vi "labbbbb.vi"() -> ()   [LabVIEW 2012]
uses:
  <vilib>/imath/engines/lvmath/Plug In/_Char/NIMS_CH_character datatype.ctl
  <vilib>/imath/engines/lvmath2/RunTimeEngine/ErrorHandling/NIMS_Finalize Error.vi
  <vilib>/imath/engines/lvmath2/RunTimeEngine/Managers/WorkSpace/UID Generator.vi
  <vilib>/imath/engines/lvmath2/RunTimeEngine/BuiltInFunctions/length/NIMS_length(GV).vi
  <instcachedir>/0/NIMS_length(GV)_08A3D13377FD4E4B96F5795FBF3698FA.lvgen/NIMS_length(GV)_08A3D13377FD4E4B96F5795FBF3698FA_002.vi
  <vilib>/imath/engines/lvmath2/RunTimeEngine/Managers/SymbolTable/Clear UID.vi
  <vilib>/imath/engines/lvmath2/RunTimeEngine/NodeEndStatement/NIMS_NodeEndStatement_Output.vi
  <instcachedir>/0/NIMS_NodeEndStatement_Output_53EC0D466D134D7ABD903AC30B43404B.lvgen/NIMS_NodeEndStatement_Output_53EC0D466D134D7ABD903AC30B43404B_011.vi
  <vilib>/imath/engines/lvmath2/RunTimeEngine/BuiltInFunctions/linramp/NIMS_linramp.vi
  <vilib>/imath/engines/lvmath2/RunTimeEngine/RangeToken/NIMS_Range_R2 - Integer.vi
  <instcachedir>/0/NIMS_Range_R2 - Integer_CD92A44154CA48D58B2F3E711AB114DB.lvgen/NIMS_Range_R2 - Integer_CD92A44154CA48D58B2F3E711AB114DB_000.vi
  <vilib>/imath/engines/lvmath2/RunTimeEngine/CommandStatement/MC_CommandStatement_break.vi
  <vilib>/imath/engines/lvmath2/RunTimeEngine/VariableToken/Read/NIMS_Get Elements - RV(_) - Check.vi
  <instcachedir>/0/NIMS_Get Elements - RV(_) - Check_09E565EE58C54071A799578B82C9999A.lvgen/NIMS_Get Elements - RV(_) - Check_09E565EE58C54071A799578B82C9999A_003.vi
  <vilib>/imathl/engines/lvmath/Functions/Error Handling/Create Error.vi
  <instcachedir>/0/NIMS_length(GV)_08A3D13377FD4E4B96F5795FBF3698FA.lvgen/NIMS_length(GV)_08A3D13377FD4E4B96F5795FBF3698FA_000.vi
  <vilib>/imath/engines/lvmath2/RunTimeEngine/BuiltInFunctions/ones/NIMS_V=ones(I32,I32).vi
  <vilib>/imath/engines/lvmath2/RunTimeEngine/RowToken/NIMS_RowToken_M_SorRV.vi
  <instcachedir>/0/NIMS_RowToken_M_SorRV_D59972FF7C1F4F35B631A72602F10CED.lvgen/NIMS_RowToken_M_SorRV_D59972FF7C1F4F35B631A72602F10CED_002.vi
  <vilib>/imath/engines/lvmath2/RunTimeEngine/BuiltInFunctions/length/NIMS_length(GM).vi
  <instcachedir>/0/NIMS_length(GM)_47CEC356FCE0482D9BA47DC61C99F2C7.lvgen/NIMS_length(GM)_47CEC356FCE0482D9BA47DC61C99F2C7_001.vi
  <vilib>/imath/engines/lvmath2/RunTimeEngine/BuiltInFunctions/figure/NIMS_figure.vi
  <vilib>/imath/engines/lvmath2/RunTimeEngine/BuiltInFunctions/subplot/NIMS_subplot(I32, I32, I32).vi
  <vilib>/imath/engines/lvmath/Plug In/_Char/NIMS_CH_Character RV to String.vi
  <vilib>/imath/engines/lvmath/Plug In/_Char/NIMS_CH_Character 1D to U8 1D.vi
  <vilib>/imath/engines/lvmath2/RunTimeEngine/RangeToken/NIMS_Range.vi
  <instcachedir>/0/NIMS_Range_3104F3C74E39439AB2C0407E7DA2F64D.lvgen/NIMS_Range_3104F3C74E39439AB2C0407E7DA2F64D_000.vi
  <vilib>/imath/engines/lvmath2/RunTimeEngine/BuiltInFunctions/plot/NIMS_plot(RM, RM, Str, Arb).vi
  <vilib>/imath/engines/lvmath2/RunTimeEngine/BuiltInFunctions/title/NIMS_title.vi
  <vilib>/imath/engines/lvmath2/RunTimeEngine/BuiltInFunctions/xlabel/NIMS_xlabel.vi
  <vilib>/imath/engines/lvmath2/RunTimeEngine/BuiltInFunctions/ylabel/NIMS_ylabel.vi
  <vilib>/imath/engines/lvmath2/RunTimeEngine/BuiltInFunctions/ylimit/NIMS_ylimit.vi
  <vilib>/imath/engines/lvmath2/RunTimeEngine/BuiltInFunctions/grid/NIMS_grid(Enums).vi
  <vilib>/imath/engines/lvmath2/RunTimeEngine/BuiltInFunctions/fft/NIMS_fft(GM).vi
  <instcachedir>/0/NIMS_fft(GM)_8E560338913F4311B445B77B8B396D1F.lvgen/NIMS_fft(GM)_8E560338913F4311B445B77B8B396D1F_000.vi
  <vilib>/imath/engines/lvmath2/RunTimeEngine/BuiltInFunctions/abs/NIMS_abs(signed).vi
  <instcachedir>/0/NIMS_abs(signed)_C4FCB8E6058B49B797C7C8D53CA5F6EC.lvgen/NIMS_abs(signed)_C4FCB8E6058B49B797C7C8D53CA5F6EC_003.vi
  <vilib>/imath/engines/lvmath2/RunTimeEngine/ErrorHandling/NIMS_Create Error From Enums.vi
  <instcachedir>/0/NIMS_length(GM)_47CEC356FCE0482D9BA47DC61C99F2C7.lvgen/NIMS_length(GM)_47CEC356FCE0482D9BA47DC61C99F2C7_000.vi
  <instcachedir>/0/NIMS_Range_3104F3C74E39439AB2C0407E7DA2F64D.lvgen/NIMS_Range_3104F3C74E39439AB2C0407E7DA2F64D_001.vi
  <vilib>/imath/engines/lvmath2/RunTimeEngine/VariableToken/Read/NIMS_Get Elements - SorM(_) - Check(_).vi
  <instcachedir>/0/NIMS_Get Elements - SorM(_) - Check(_)_2E5C1E1F82C046EDA67048B0831F877E.lvgen/NIMS_Get Elements - SorM(_) - Check(_)_2E5C1E1F82C046EDA67048B0831F877E_008.vi
  <vilib>/imath/engines/lvmath2/RunTimeEngine/BuiltInFunctions/plot/NIMS_plot(RM, RM, Str).vi
  <vilib>/imath/engines/lvmath2/RunTimeEngine/RunTimeType/NIMS_RunTimeType_From StrictType (excl LVString).vi
  <instcachedir>/0/NIMS_RunTimeType_From StrictType (excl LVString)_AC52D965D0864706932D20A05968E122.lvgen/NIMS_RunTimeType_From StrictType (excl LVString)_AC52D965D0864706932D20A05968E122_001.vi
  <vilib>/imath/engines/lvmath2/RunTimeEngine/LocalVariableDefStatement/MC_LocalVariableDefStatement_Display.vi
  <vilib>/imath/engines/lvmath2/RunTimeEngine/BuiltInFunctions/num_to_str/NIMS_num_to_str(GRowV,I32).vi
  <instcachedir>/0/NIMS_num_to_str(GRowV,I32)_1267845AD1B74D9CA82282F86654A6BA.lvgen/NIMS_num_to_str(GRowV,I32)_1267845AD1B74D9CA82282F86654A6BA_000.vi
  <vilib>/imath/engines/lvmath/Plug In/_Char/NIMS_CH_String to Character Array.vi
  <vilib>/imath/engines/lvmath2/RunTimeEngine/ErrorHandling/NIMS_Error From Error Code.vi
  <vilib>/imath/engines/lvmath2/RunTimeEngine/Managers/SymbolTable/NIMS_WorkSpace.lvlib
panel:
  out "Polar Biphase":i32[][](graph)
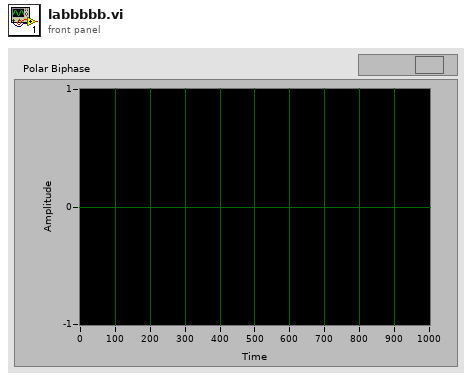
[diagram p1: front panel]
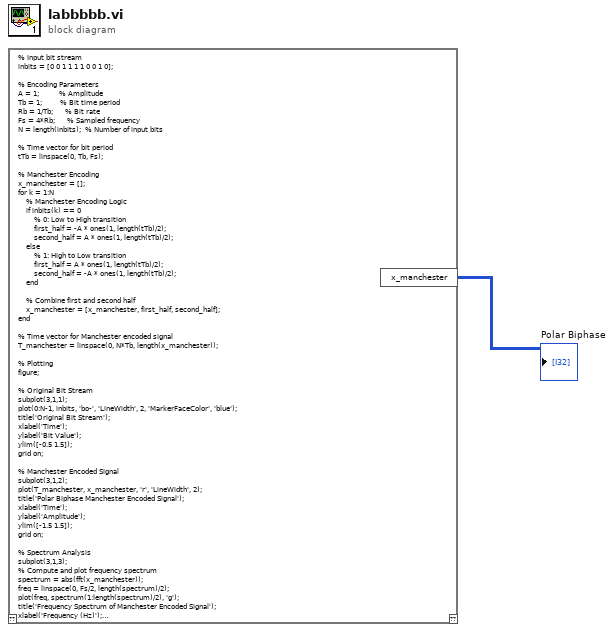
[diagram p0: block diagram]
diagram:
  n1 = mathscript code="% Input bit stream\ninbits = [0 0 1 1 1 1 0 0 1 0];\n\n% Encoding Parameters\nA = 1;          % Amplitude\nTb = 1;         % Bit time period\nRb = 1/Tb;      % Bit rate\nFs = 4*Rb;      % Sampled frequency\nN = length(inbits);  % Number of input bits\n\n% Time vector for bit period\ntTb = linspace(0, Tb, Fs);\n\n% Manchester Encoding\nx_manchester = [];\nfor k = 1:N\n    % Manchester Encoding Logic\n    if inbits(k) == 0\n        % 0: Low to High transition\n        first_half = -A * ones(1, length(tTb)/2);\n        second_half = A * ones(1, length(tTb)/2);\n    else\n        % 1: High to Low transition\n        first_half = A * ones(1, length(tTb)/2);\n        second_half = -A * ones(1, length(tTb)/2);\n    end\n    \n    % Combine first and second half\n    x_manchester = [x_manchester, first_half, second_half];\nend\n\n% Time vector for Manchester encoded signal\nT_manchester = linspace(0, N*Tb, length(x_manchester));\n\n% Plotting\nfigure;\n\n% Original Bit Stream\nsubplot(3,1,1);\nplot(0:N-1, inbits, 'bo-', 'LineWidth', 2, 'MarkerFaceColor', 'blue');\ntitle('Original Bit Stream');\nxlabel('Time');\nylabel('Bit Value');\nylim([-0.5 1.5]);\ngrid on;\n\n% Manchester Encoded Signal\nsubplot(3,1,2);\nplot(T_manchester, x_manchester, 'r', 'LineWidth', 2);\ntitle('Polar Biphase Manchester Encoded Signal');\nxlabel('Time');\nylabel('Amplitude');\nylim([-1.5 1.5]);\ngrid on;\n\n% Spectrum Analysis\nsubplot(3,1,3);\n% Compute and plot frequency spectrum\nspectrum = abs(fft(x_manchester));\nfreq = linspace(0, Fs/2, length(spectrum)/2);\nplot(freq, spectrum(1:length(spectrum)/2), 'g');\ntitle('Frequency Spectrum of Manchester Encoded Signal');\nxlabel('Frequency (Hz)');\nylabel('Magnitude');\ngrid on;\n\n% Print signal characteristics\ndisp('Manchester Encoded Signal Characteristics:');\ndisp(['Signal Length: ', num2str(length(x_manchester))]);\ndisp(['Peak Amplitude: ±', num2str(A)]);\ndisp(['Bit Duration: ', num2str(Tb), ' seconds']);\ndisp(['Sampling Frequency: ', num2str(Fs), ' Hz']);"() -> ("x_manchester"=→"Polar Biphase":i32[][])  [unwired: 1 in, 1 out]
